vi "fgv_PwrPak7-data.vi"(7 "cmd":T2, 8 "error in":errorcluster, 11 "data cluster in":T1={"rawdata"="", "GPS Data"={"Latitude"={"Valid?"=TRUE, "Latitude (Deg)"=37.37123095061}, "Longitude"={"Valid?"=TRUE, "Longitude (Deg)"=126.72256864175}, "Height"={"Valid?"=TRUE, "Height (m)"=9.9059}, "Undulation"={"Valid?"=TRUE, "Undulation(m)"=22.3}, "North Vel"={"Valid?"=TRUE, "North Vel (m/s)"=-0.0013}, "East Vel"={"Valid?"=TRUE, "East Vel (m/s)"=-0.002}, "Up Vel"={"Valid?"=TRUE, "Up Vel (m/s)"=0.0004}, "Roll"={"Valid?"=TRUE, "Roll (degrees)"=-0.425709275}, "Pitch"={"Valid?"=TRUE, "Pitch (degrees)"=-0.898393069}, "Azimuth"={"Valid?"=TRUE, "Azimuth (degrees)"=98.594488749}, "Lat deviation"={"Valid?"=TRUE, "Lat deviation (m)"=0.4755}, "Long deviation"={"Valid?"=TRUE, "Long deviation (m)"=0.4754}, "Height deviation"={"Valid?"=TRUE, "Height deviation (m)"=0.9034}, "North vel deviation"={"Valid?"=TRUE, "North vel deviation (m/s)"=0.0181}, "East vel deviation"={"Valid?"=TRUE, "East vel deviation (m/s)"=0.018}, "Up vel deviation"={"Valid?"=TRUE, "Up vel deviation (m/s)"=0.0196}, "Roll deviation"={"Valid?"=TRUE, "Roll deviation (degrees)"=0.0309}, "Pitch deviation"={"Valid?"=TRUE, "Pitch deviation (degrees)"=0.0311}, "Azimuth deviation"={"Valid?"=TRUE, "Azimuth deviation (degrees)"=0.1368}, "Ext sol status"={"Valid?"=TRUE, "Ext sol status"=0.0}}, "Heading"=98.684623718, "utm-1"={"XN"=530126.7583503594, "YE"=175270.68061157822}} {"utm-1"."XN" format="%.2f"; "utm-1"."YE" format="%.2f"}) -> (0 "error out":errorcluster, 3 "data cluster out":T1={"rawdata"="", "GPS Data"={"Latitude"={"Valid?"=TRUE, "Latitude (Deg)"=37.37123095061}, "Longitude"={"Valid?"=TRUE, "Longitude (Deg)"=126.72256864175}, "Height"={"Valid?"=TRUE, "Height (m)"=9.9059}, "Undulation"={"Valid?"=TRUE, "Undulation(m)"=22.3}, "North Vel"={"Valid?"=TRUE, "North Vel (m/s)"=-0.0013}, "East Vel"={"Valid?"=TRUE, "East Vel (m/s)"=-0.002}, "Up Vel"={"Valid?"=TRUE, "Up Vel (m/s)"=0.0004}, "Roll"={"Valid?"=TRUE, "Roll (degrees)"=-0.425709275}, "Pitch"={"Valid?"=TRUE, "Pitch (degrees)"=-0.898393069}, "Azimuth"={"Valid?"=TRUE, "Azimuth (degrees)"=98.594488749}, "Lat deviation"={"Valid?"=TRUE, "Lat deviation (m)"=0.4755}, "Long deviation"={"Valid?"=TRUE, "Long deviation (m)"=0.4754}, "Height deviation"={"Valid?"=TRUE, "Height deviation (m)"=0.9034}, "North vel deviation"={"Valid?"=TRUE, "North vel deviation (m/s)"=0.0181}, "East vel deviation"={"Valid?"=TRUE, "East vel deviation (m/s)"=0.018}, "Up vel deviation"={"Valid?"=TRUE, "Up vel deviation (m/s)"=0.0196}, "Roll deviation"={"Valid?"=TRUE, "Roll deviation (degrees)"=0.0309}, "Pitch deviation"={"Valid?"=TRUE, "Pitch deviation (degrees)"=0.0311}, "Azimuth deviation"={"Valid?"=TRUE, "Azimuth deviation (degrees)"=0.1368}, "Ext sol status"={"Valid?"=TRUE, "Ext sol status"=0.0}}, "Heading"=98.684623718, "utm-1"={"XN"=530126.7583503594, "YE"=175270.68061157822}} {"utm-1"."XN" format="%.2f"; "utm-1"."YE" format="%.2f"})   [LabVIEW 2019]
uses:
  Ctrl/gps-databuf.ctl
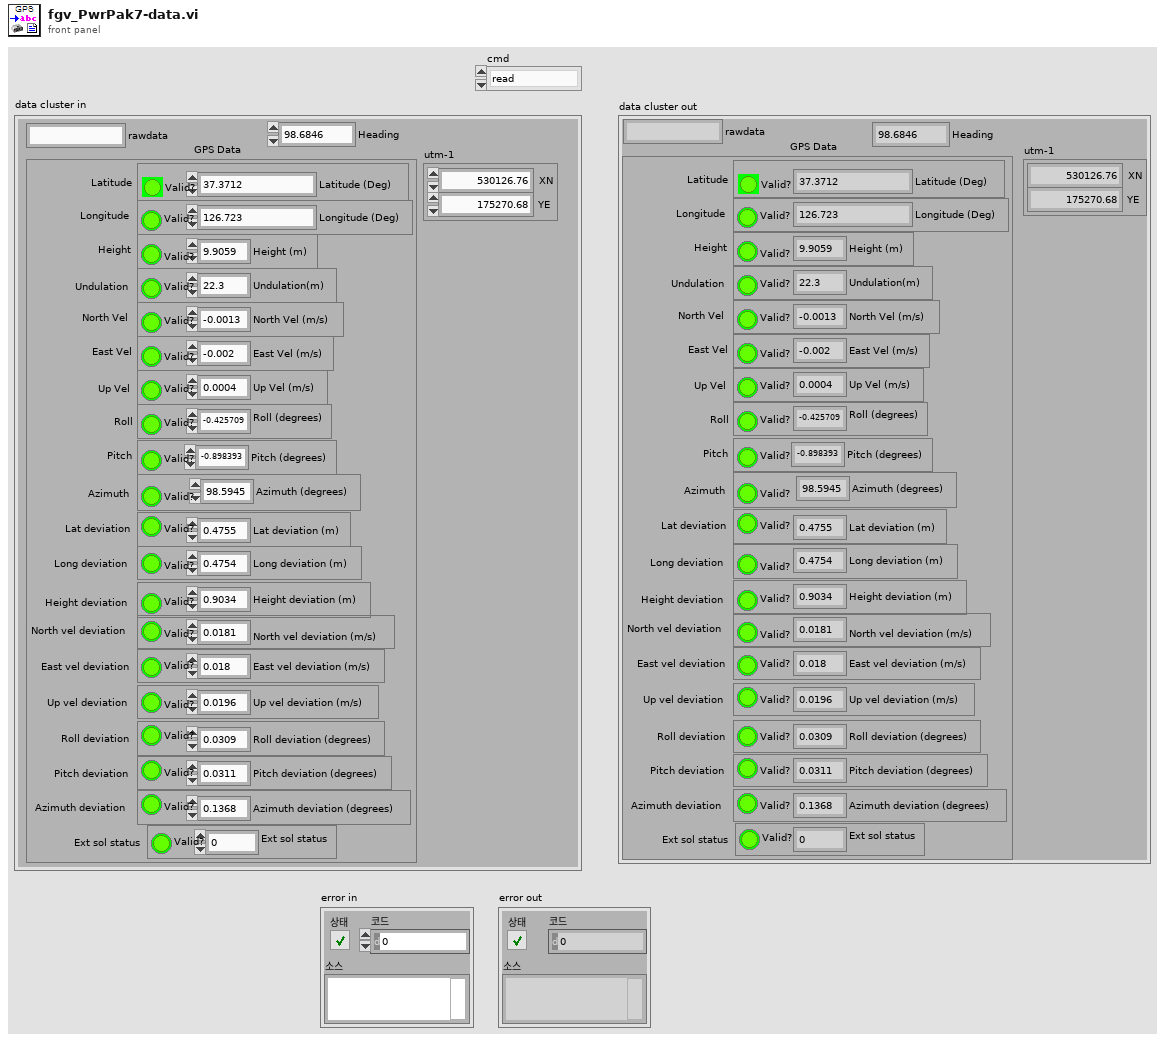
[diagram p1: front panel]
types:
  T1 = cluster{"rawdata":string, "GPS Data":cluster{"Latitude":cluster{"Valid?":bool, "Latitude (Deg)":dbl}, "Longitude":cluster{"Valid?":bool, "Longitude (Deg)":dbl}, "Height":cluster{"Valid?":bool, "Height (m)":dbl}, "Undulation":cluster{"Valid?":bool, "Undulation(m)":dbl}, "North Vel":cluster{"Valid?":bool, "North Vel (m/s)":dbl}, "East Vel":cluster{"Valid?":bool, "East Vel (m/s)":dbl}, "Up Vel":cluster{"Valid?":bool, "Up Vel (m/s)":dbl}, "Roll":cluster{"Valid?":bool, "Roll (degrees)":dbl}, "Pitch":cluster{"Valid?":bool, "Pitch (degrees)":dbl}, "Azimuth":cluster{"Valid?":bool, "Azimuth (degrees)":dbl}, "Lat deviation":cluster{"Valid?":bool, "Lat deviation (m)":dbl}, "Long deviation":cluster{"Valid?":bool, "Long deviation (m)":dbl}, "Height deviation":cluster{"Valid?":bool, "Height deviation (m)":dbl}, "North vel deviation":cluster{"Valid?":bool, "North vel deviation (m/s)":dbl}, "East vel deviation":cluster{"Valid?":bool, "East vel deviation (m/s)":dbl}, "Up vel deviation":cluster{"Valid?":bool, "Up vel deviation (m/s)":dbl}, "Roll deviation":cluster{"Valid?":bool, "Roll deviation (degrees)":dbl}, "Pitch deviation":cluster{"Valid?":bool, "Pitch deviation (degrees)":dbl}, "Azimuth deviation":cluster{"Valid?":bool, "Azimuth deviation (degrees)":dbl}, "Ext sol status":cluster{"Valid?":bool, "Ext sol status":dbl}}, "Heading":dbl, "utm-1":cluster{"XN":dbl, "YE":dbl}}
  T2 = typedef "gps-databuf.ctl" = enum16{"read", "write"}
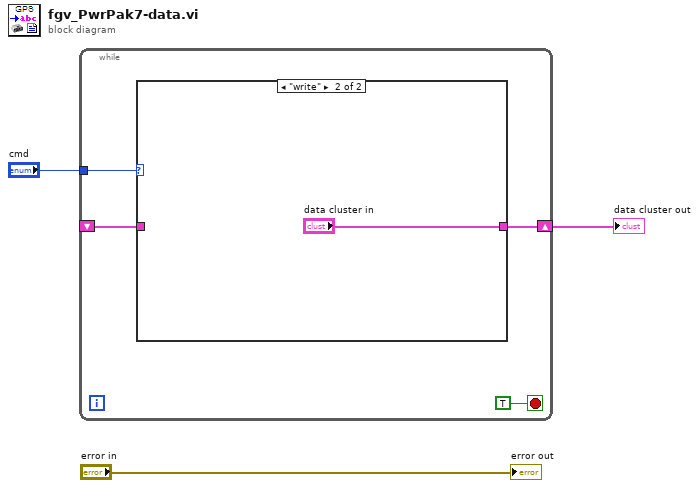
[diagram p0: block diagram]
diagram:
  n1 = while {
    tunnel: "cmd" -> [w6]
    shift-right: [w5] -> w2
    shift-left: _ -> [w4]
    stop <- TRUE stop-if-true
    n2 = case shown="\"write\"" w6 {
      tunnel: [w8 "data cluster in"] -> w5
      tunnel: w4 -> [w8 _]
      frame "read", Default {
      }
      frame "write" {
      }
    }
  }
  "data cluster out" <- w2
  "error out" <- "error in"
